vi "LOGNPAGE.vi"() -> ()   [LabVIEW 2018]
panel:
  in  "Tab Control":enum32{"Page 1", "Page 2"}(tab)
  in  "Exit":bool caption="Enter"
  in  "Enter":bool
  in  "Nume":string
  in  "Parola":string
  in  "Login":bool
  in  "Reset":bool
  in  "Close":bool
  # "Bun venit la aplicatie data-loggin in labview (File I / O)"
  # "De Baloi Razvan"
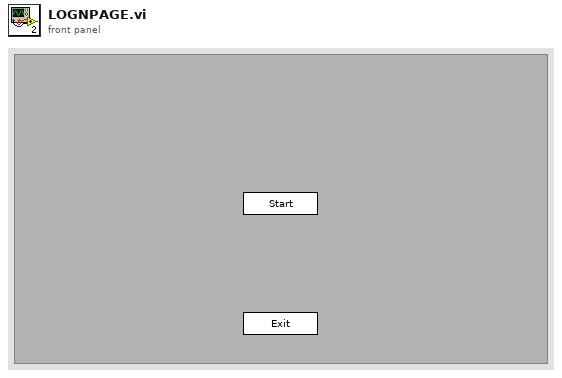
[diagram p1: front panel]
types:
  T1 = enum32{"Invalid", "Standard", "Closed", "Hidden", "Minimized", "Maximized"}
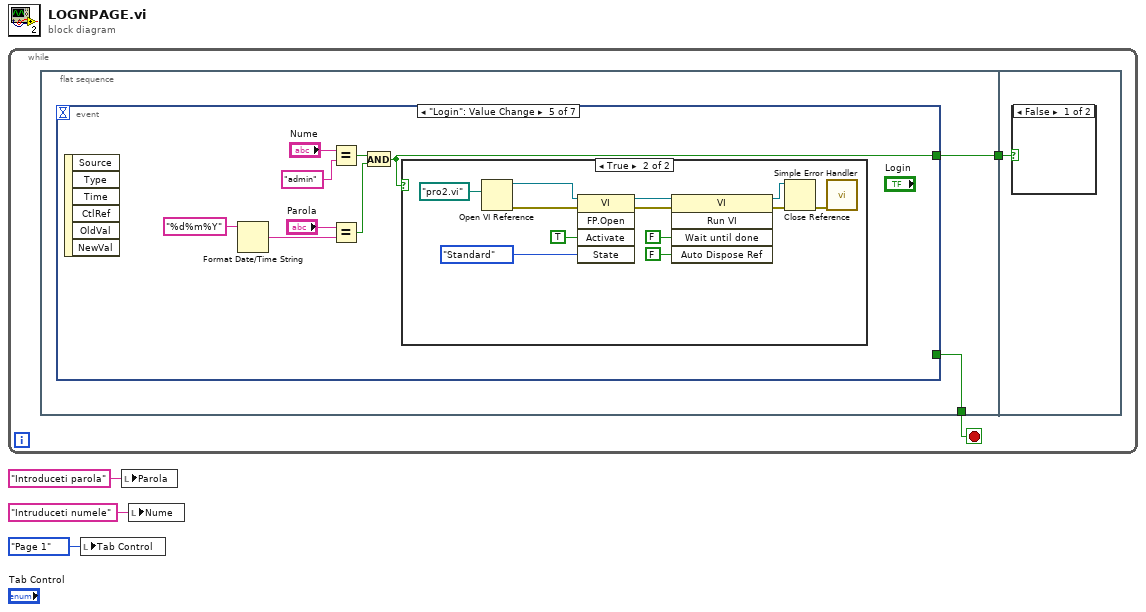
[diagram p0: block diagram]
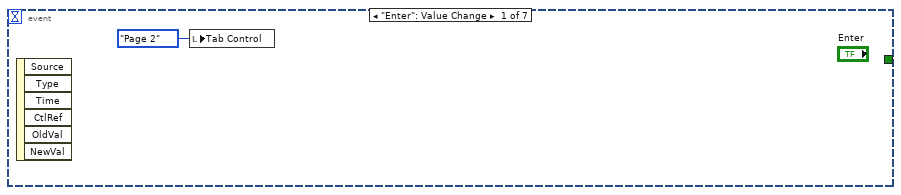
[diagram p2: hidden frame]
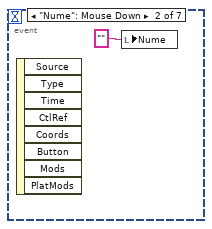
[diagram p3: hidden frame]
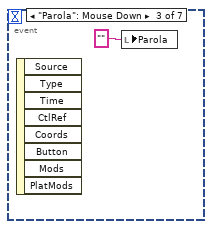
[diagram p4: hidden frame]
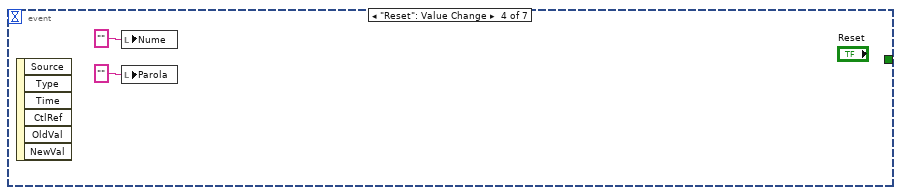
[diagram p5: hidden frame]
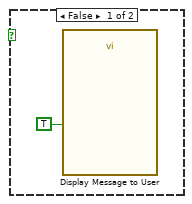
[diagram p6: hidden frame]
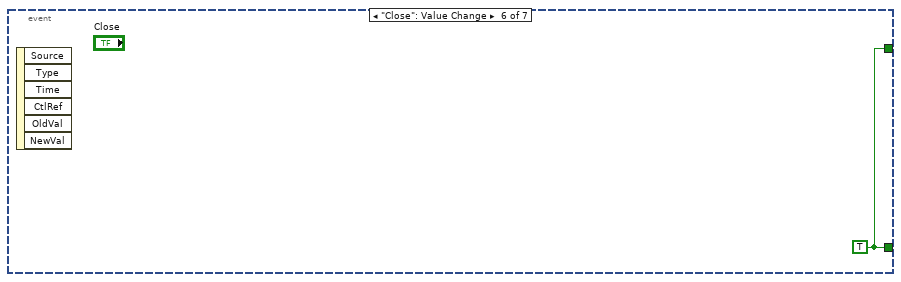
[diagram p7: hidden frame]
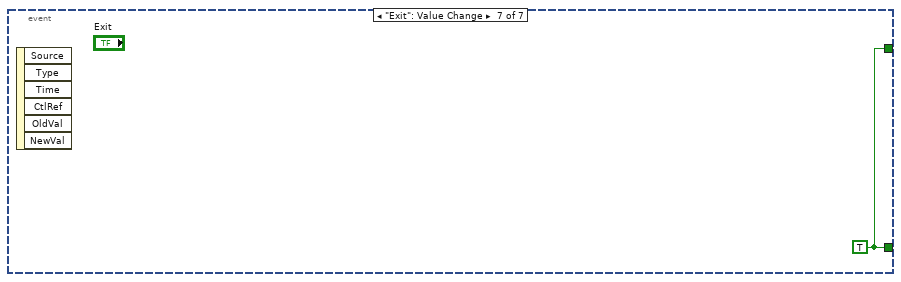
[diagram p8: hidden frame]
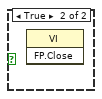
[diagram p9: hidden frame]
diagram:
  n1 = while {
    stop <- w4 stop-if-true
    n2 = flat-sequence {
      tunnel: [w7] -> w5
      tunnel: [w6] -> w4
      tunnel: w5 -> [w36]
      frame #0 {
        n3 = event shown="[4] \"Login\": Value Change" {
          selector: _ -> [_ _ _ _ _ _ _]
          dyn-events: _ -> [_ _ _ _ _ _ _]
          timeout: _ -> [_ _ _ _ _ _ _]
          tunnel: [_ _ _ _ w13 w34 w35] -> w7
          tunnel: [_ _ _ _ _ w34 w35] -> w6
          event "Enter": Value Change {
            n4 = event-data() -> ()  [unwired: 1 in, 6 out]
            n5 = local write "Tab Control"(enum32{"Page 1", "Page 2"}."Page 2" ("Tab Control")) -> ()
          }
          event "Nume": Mouse Down {
            n6 = event-data() -> ()  [unwired: 1 in, 8 out]
            n7 = local write "Nume"("" ("Nume")) -> ()
          }
          event "Parola": Mouse Down {
            n8 = event-data() -> ()  [unwired: 1 in, 8 out]
            n9 = local write "Parola"("" ("Parola")) -> ()
          }
          event "Reset": Value Change {
            n10 = event-data() -> ()  [unwired: 1 in, 6 out]
            n11 = local write "Nume"("" ("Nume")) -> ()
            n12 = local write "Parola"("" ("Parola")) -> ()
          }
          event "Login": Value Change {
            n13 = event-data() -> ()  [unwired: 1 in, 6 out]
            n14 = Format Date/Time String(time format string (%c)="%d%m%Y") -> (date/time string=w16:string)  [unwired: 2 in]
            n15 = Equal?(x="Nume", y="admin") -> (x = y?=w14:bool)
            n16 = Equal?(x="Parola", y=w16) -> (x = y?=w15:bool)
            n17 = And(x=w14, y=w15) -> (x .and. y?=w13:bool)
            n18 = case shown="True" w13 {
              frame False {
                n19 = call "Display Message to User"("Enable"=TRUE) -> ()  [unwired: 9 in, 2 out]
              }
              frame True {
                n20 = Open VI Reference(vi path=path "pro2.vi") -> (vi reference=w32:refnum<vi>, error out=w31:errorcluster)  [unwired: 5 in]
                n21 = invoke class="VI" method="FP.Open"(reference=w32, error in=w31, "Activate"=TRUE ("Activate?"), "State"=T1."Standard") -> (reference out=w30:refnum<vi>, error out=w29:errorcluster)  [unwired: 1 in, 3 out]
                n22 = invoke class="VI" method="Run VI"(reference=w30, error in=w29, "Wait until done"=FALSE ("Wait Until Done"), "Auto Dispose Ref"=FALSE ("Auto Dispose Reference")) -> (reference out=w24:refnum<vi>, error out=w23:errorcluster)  [unwired: 1 in, 3 out]
                n23 = Close Reference(reference=w24, error in (no error)=w23) -> (error out=w22:errorcluster)
                n24 = call <vilib>:"Simple Error Handler.vi"("error in (no error)"=w22) -> ()  [unwired: 4 in, 5 out]
              }
            }
          }
          event "Close": Value Change {
            w34 = TRUE
            n25 = event-data() -> ()  [unwired: 1 in, 6 out]
          }
          event "Exit": Value Change {
            w35 = TRUE
            n26 = event-data() -> ()  [unwired: 1 in, 6 out]
          }
        }
      }
      frame #1 {
        n27 = case shown="False" w36 {
          frame False {
          }
          frame True {
            n28 = invoke class="VI" method="FP.Close"() -> ()  [unwired: 3 in, 3 out]
          }
        }
      }
    }
  }
  n29 = local write "Tab Control"(enum32{"Page 1", "Page 2"}."Page 1" ("Tab Control")) -> ()
  n30 = local write "Parola"("Introduceti parola" ("Parola")) -> ()
  n31 = local write "Nume"("Intruduceti numele" ("Nume")) -> ()
